vi "Get Wheel Colors.vi"(8 "error in (no error)":errorcluster, 11 "dialog info in":T1={"steering frame ref"=refnum, "active wheel indexes"=[], "FP Refs"={"VI Refnum"=refnum, "Menu Ref"=refnum, "Sub Panel"=refnum, "picture"=refnum, "Steering Type"=refnum, "zoom in"=refnum, "zoom out"=refnum, "zoom extents"=refnum, "Wheels"=refnum, "Add Wheel"=refnum, "Remove Wheel"=refnum, "Copy Wheel"=refnum, "Angle Units"=refnum}, "subpanel info"={"subpanel VI refs"=[], "subpanel types"=[], "main to subpanel command events"=[]}, "picture dragging state"={"dragging"=FALSE, "wheel index"=-1, "dragging mode"=enum."translate", "wheel start position"={"x"=0.0, "y"=0.0, "theta"=0.0}, "relative mouse position"={"x"=0.0, "y"=0.0}, "relative mouse init angle (rad)"=0.0}, "picture size (pixels)"={"Width"=500, "Height"=500}, "picture grid"=bytes[0], "click zones group"={"click zones array"=[], "num click zones"=0}, "draw options"={"draw wheel states?"=FALSE, "highlight wheel index"=-1, "pixels per unit"=10.0, "draw forward velocity?"=FALSE, "velocity scale"=1.0}}) -> (0 "error out":errorcluster, 2 "wheel colors":u32[](array[colorbox]), 3 "dialog info out":T1={"steering frame ref"=refnum, "active wheel indexes"=[], "FP Refs"={"VI Refnum"=refnum, "Menu Ref"=refnum, "Sub Panel"=refnum, "picture"=refnum, "Steering Type"=refnum, "zoom in"=refnum, "zoom out"=refnum, "zoom extents"=refnum, "Wheels"=refnum, "Add Wheel"=refnum, "Remove Wheel"=refnum, "Copy Wheel"=refnum, "Angle Units"=refnum}, "subpanel info"={"subpanel VI refs"=[], "subpanel types"=[], "main to subpanel command events"=[]}, "picture dragging state"={"dragging"=FALSE, "wheel index"=-1, "dragging mode"=enum."translate", "wheel start position"={"x"=0.0, "y"=0.0, "theta"=0.0}, "relative mouse position"={"x"=0.0, "y"=0.0}, "relative mouse init angle (rad)"=0.0}, "picture size (pixels)"={"Width"=500, "Height"=500}, "picture grid"=bytes[0], "click zones group"={"click zones array"=[], "num click zones"=0}, "draw options"={"draw wheel states?"=FALSE, "highlight wheel index"=-1, "pixels per unit"=10.0, "draw forward velocity?"=FALSE, "velocity scale"=1.0}})   [LabVIEW 2017, in "NI_Robotics_Configure Steering Frame.lvlib"]
uses:
  <vilib>/robotics/Dialog/Configure Steering Frame/NI_Robotics_Configure Steering Frame.lvlib
  <vilib>/robotics/Dialog/Configure Steering Frame/Dialog Info.ctl
  <vilib>/robotics/Steering/Steering Frame/NI_Robotics_Steering Frame.lvclass
  <vilib>/robotics/Dialog/Configure Steering Frame/FP Refs.ctl
  <vilib>/robotics/Dialog/Configure Steering Frame/Subpanel Info.ctl
  <vilib>/robotics/Dialog/Configure Steering Frame/Main to Subpanel Command Event.ctl
  <vilib>/robotics/Dialog/Configure Steering Frame/Main to Subpanel Command.ctl
  <vilib>/robotics/Dialog/Configure Steering Frame/Dragging State.ctl
  <vilib>/robotics/Dialog/Configure Steering Frame/Dragging Mode.ctl
  <vilib>/Utility/miscctls.llb/LVBoundsTypeDef.ctl
  <vilib>/robotics/Dialog/Configure Steering Frame/Click Zone.ctl
  <vilib>/robotics/Utilities/Visualization/Steering Visualization/Steering Picture/Draw Steering Frame Options.ctl
  <vilib>/robotics/Steering/Steering Frame/NI_Robotics_Steering Frame.lvclass/NI_Robotics_Steering Frame.ctl
  <vilib>/robotics/Utilities/Visualization/Steering Visualization/Steering Picture/NI_Robotics_Steering Picture.lvlib
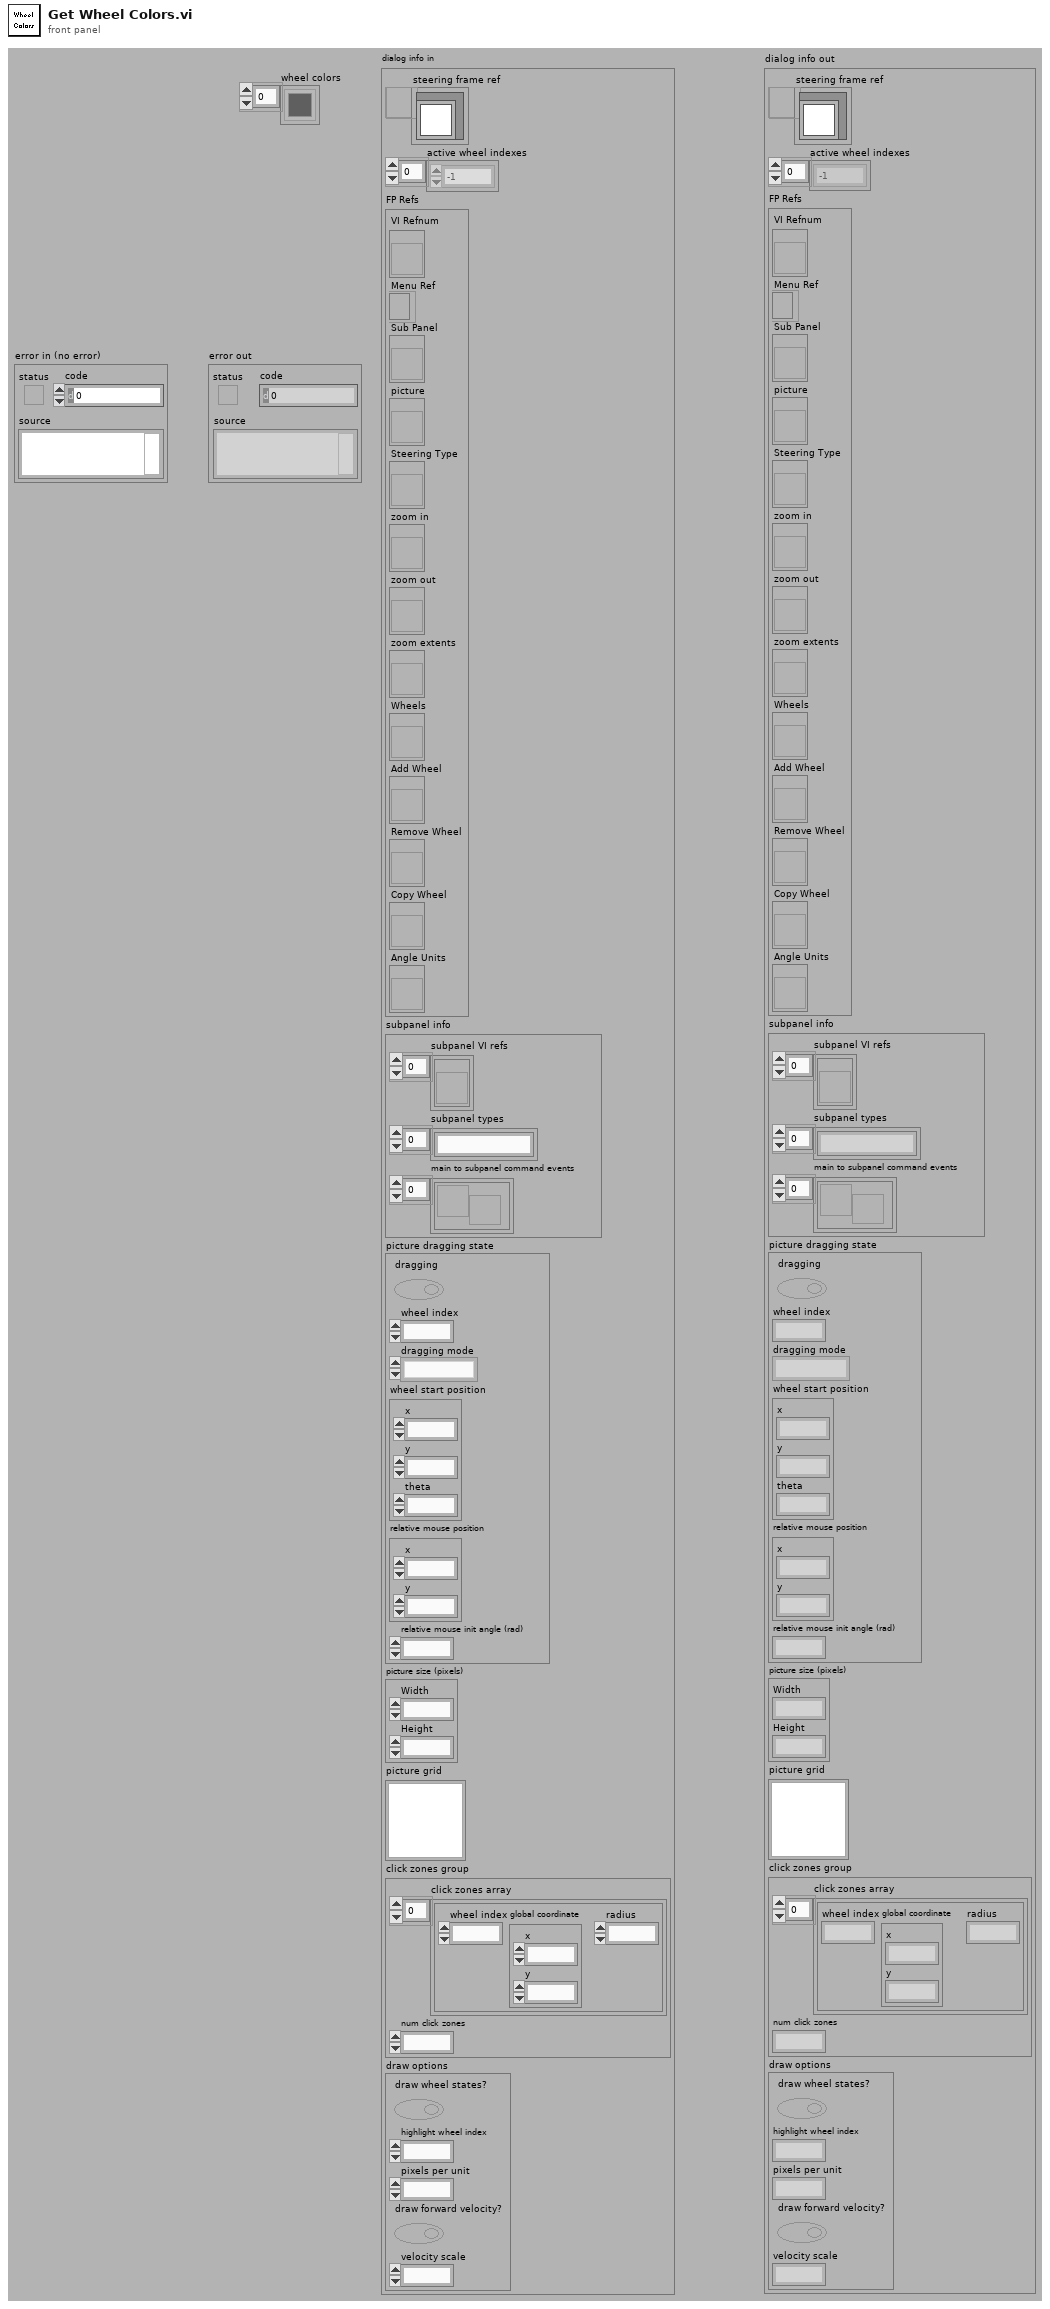
[diagram p1: front panel]
types:
  T1 = typedef "NI_Robotics_Configure Steering Frame.lvlib/Dialog Info.ctl" = cluster{"steering frame ref":refnum<data-value>, "active wheel indexes":i32[], "FP Refs":T2, "subpanel info":T3, "picture dragging state":T5, "picture size (pixels)":T7, "picture grid":picture, "click zones group":cluster{"click zones array":T8[], "num click zones":i32}, "draw options":T9}
  T2 = typedef "NI_Robotics_Configure Steering Frame.lvlib/FP Refs.ctl" = cluster{"VI Refnum":refnum<vi>, "Menu Ref":refnum<k9>, "Sub Panel":refnum<vi>, "picture":refnum<vi>, "Steering Type":refnum<vi>, "zoom in":refnum<vi>, "zoom out":refnum<vi>, "zoom extents":refnum<vi>, "Wheels":refnum<vi>, "Add Wheel":refnum<vi>, "Remove Wheel":refnum<vi>, "Copy Wheel":refnum<vi>, "Angle Units":refnum<vi>}
  T3 = typedef "NI_Robotics_Configure Steering Frame.lvlib/Subpanel Info.ctl" = cluster{"subpanel VI refs":refnum<vi>[], "subpanel types":string[], "main to subpanel command events":T4[]}
  T4 = typedef "NI_Robotics_Configure Steering Frame.lvlib/Main to Subpanel Command Event.ctl" = refnum<user-event>
  T5 = typedef "NI_Robotics_Configure Steering Frame.lvlib/Dragging State.ctl" = cluster{"dragging":bool, "wheel index":i32, "dragging mode":T6, "wheel start position":cluster{"x":dbl, "y":dbl, "theta":dbl}, "relative mouse position":cluster{"x":dbl, "y":dbl}, "relative mouse init angle (rad)":dbl}
  T6 = typedef "NI_Robotics_Configure Steering Frame.lvlib/Dragging Mode.ctl" = enum16{"translate", "rotate"}
  T7 = typedef "LVBoundsTypeDef.ctl" = cluster{"Width":u32, "Height":u32}
  T8 = typedef "NI_Robotics_Configure Steering Frame.lvlib/Click Zone.ctl" = cluster{"wheel index":i32, "global coordinate":cluster{"x":dbl, "y":dbl}, "radius":dbl}
  T9 = typedef "NI_Robotics_Steering Picture.lvlib/Draw Steering Frame Options.ctl" = cluster{"draw wheel states?":bool, "highlight wheel index":i32, "pixels per unit":dbl, "draw forward velocity?":bool, "velocity scale":dbl}
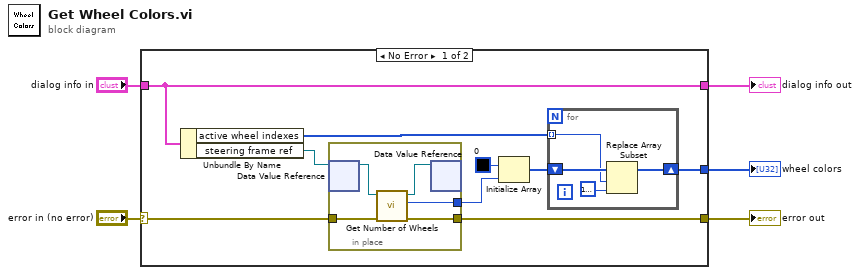
[diagram p0: block diagram]
diagram:
  n1 = case shown="No Error" "error in (no error)" {
    selector: "error in (no error)" -> [w12 w25]
    tunnel: "dialog info in" -> [w13 w24]
    tunnel: [w9 w25] -> w3
    tunnel: [w13 w24] -> w2
    tunnel: [w6 _] -> w1
    frame No Error {
      n2 = Unbundle By Name(w13) -> ("active wheel indexes"=w8:i32[], "steering frame ref"=w14:refnum<data-value>)
      n3 = in-place {
        in-place-border: w12 -> [w21]
        in-place-border: [w20] -> w9
        in-place-border: [w19] -> w11
        n4 = in-place-dvr #1(w14) -> (w23:refnum<class "NI_Robotics_Steering Frame.lvclass">)  [unwired: 1 out]
        n5 = call <vilib>:"Get Number of Wheels.vi"("error in (no error)"=w21, "steering frame in"=w23) -> ("error out"=w20:errorcluster, "number of wheels"=w19:i32, "steering frame out"=w22:refnum<class "NI_Robotics_Steering Frame.lvclass">)  [unwired: 7 in]
        n6 = in-place-dvr #1(w22) -> ()  [unwired: 2 out]
      }
      n7 = Initialize Array(u32 0, w11) -> (w7:u32[])
      n8 = for {
        tunnel: w8 -> [w16] mode=indexing
        shift-right: [w17] -> w6
        shift-left: w7 -> [w18]
        n9 = Replace Array Subset(array=w18, new element=u32 16777224 ("color (black)"), index=w16) -> (w17:u32[])
      }
    }
    frame Error {
    }
  }
  "dialog info out" <- w2
  "error out" <- w3
  "wheel colors" <- w1
